vi "P4CMD Uninitialize.vi"(8 "error in (no error)":errorcluster) -> (0 "error out":errorcluster)   [LabVIEW 2020, in "NI_SCC_P4CMD.lvlib"]
uses:
  <vilib>/SourceControl/Providers/P4CMD/NI_SCC_P4CMD.lvlib
  <vilib>/SourceControl/Providers/P4CMD/P4CMD Mgr Functions.ctl
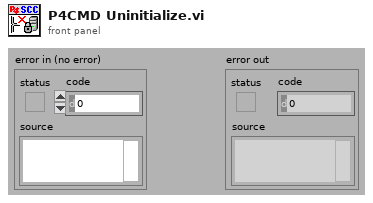
[diagram p1: front panel]
types:
  T1 = typedef "NI_SCC_P4CMD.lvlib/P4CMD Mgr Functions.ctl" = enum16{"Init", "Open", "Set Config Opts", "Initialized?", "IsRefValid?", "Get Config Opts", "Get Global Commands", "Close", "Uninit"}
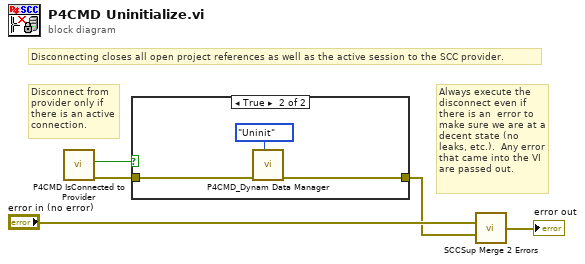
[diagram p0: block diagram]
diagram:
  # "Always execute the disconnect even if there is an  error to make sure we are at a decent state (no leaks, etc.).  Any error that came into the VI are passed out."
  # "Disconnecting closes all open project references as well as the active session to the SCC provider."
  # "Disconnect from provider only if there is an active connection."
  n1 = call <vilib>:"P4CMD IsConnected to Provider.vi"() -> ("error out"=w4:errorcluster, "active connection?"=w5:bool)  [unwired: 10 in]
  n2 = case shown="True" w5 {
    tunnel: w4 -> [w6 w9]
    tunnel: [w6 w7] -> w2
    frame False {
    }
    frame True {
      n3 = call <vilib>:"P4CMD_Dynam Data Manager.vi"("function"=P4CMD_Mgr_Functions."Uninit", "error in (no error)"=w9) -> ("error out"=w7:errorcluster)  [unwired: 4 in, 5 out]
    }
  }
  n4 = call <vilib>:"SCCSup Merge 2 Errors.vi"("Error IO 1"="error in (no error)", "Error IO 2"=w2) -> ("Error IO out"=→"error out":errorcluster)  [unwired: 13 in]
